vi "Initialize.vi"(8 "error in (no error)":errorcluster, 10 "Ctl Refnum":refnum<vi>, 11 "Pane Object Position in":refnum<class "Pane Object Position.lvclass">) -> (0 "error out":errorcluster, 3 "Pane Object Position out":refnum<class "Pane Object Position.lvclass">)   [LabVIEW 2018, in "Pane Object Position.lvclass"]
uses:
  Pane Object Position.lvclass
  Pane Object Position.lvclass/Pane Object Position.ctl
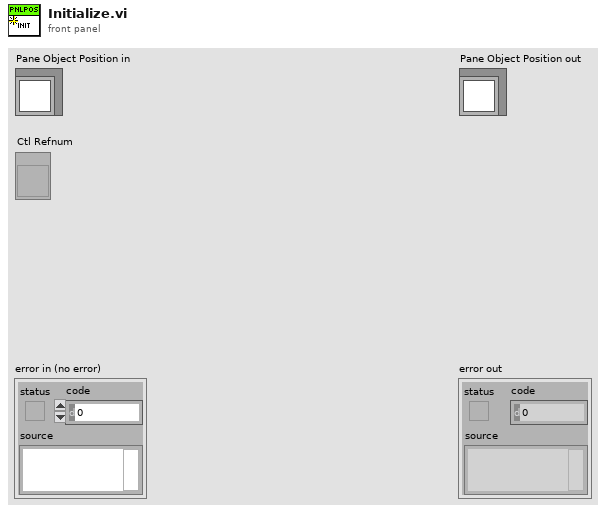
[diagram p1: front panel]
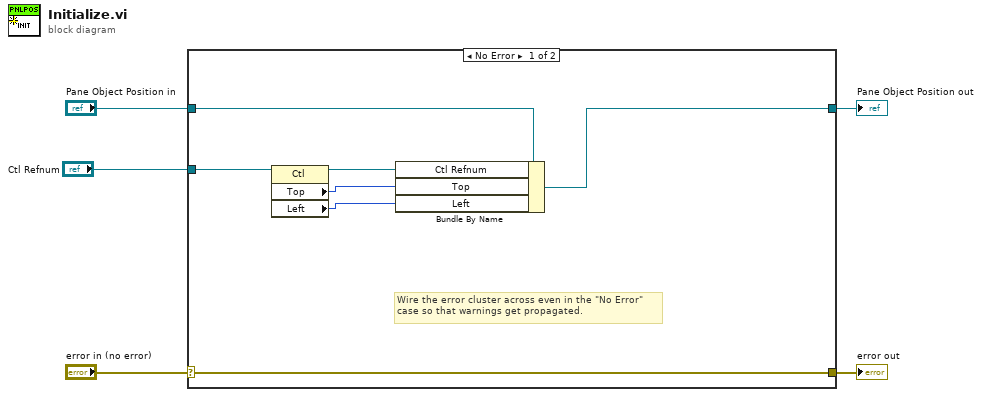
[diagram p0: block diagram]
diagram:
  n1 = case shown="No Error" "error in (no error)" {
    selector: "error in (no error)" -> [w12 w14]
    tunnel: [w12 w14] -> w4
    tunnel: [w6 w13] -> w2
    tunnel: "Pane Object Position in" -> [w10 w13]
    tunnel: "Ctl Refnum" -> [w11 _]
    frame No Error {
      # "Wire the error cluster across even in the \"No Error\"\ncase so that warnings get propagated."
      n2 = property class="Ctl"(reference=w11) -> (reference out=w9:refnum<vi>, "Top"=w8:i32, "Left"=w7:i32)  [unwired: 1 in, 1 out]
      n3 = Bundle By Name(cluster=w10, "Ctl Refnum"=w9, "Top"=w8, "Left"=w7) -> (w6:refnum<class "Pane Object Position.lvclass">)
    }
    frame Error {
    }
  }
  "error out" <- w4
  "Pane Object Position out" <- w2
